vi "Enter.vi"(8 "error in (no error)":errorcluster, 10 "User Input":string, 11 "ATM Controller in":refnum<class "ATM Controller.lvclass">) -> (0 "error out":errorcluster, 3 "ATM Controller out":refnum<class "ATM Controller.lvclass">)   [LabVIEW 2020, in "ATM Controller.lvclass"]
uses:
  ATM Controller.lvclass
  ATM Controller.lvclass/ATM Controller.ctl
  Account Database/Account Database.lvclass
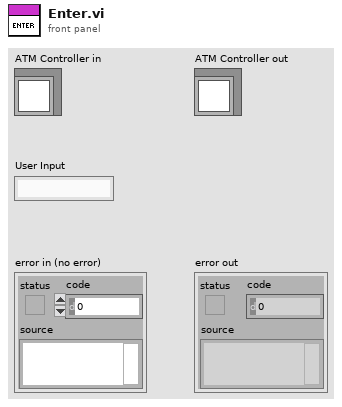
[diagram p1: front panel]
types:
  T1 = typedef "ATM Controller.lvclass/State.ctl" = enum16{"Start", "Card Inserted", "Verification Failed", "Verification Succeeded", "Terminate"}
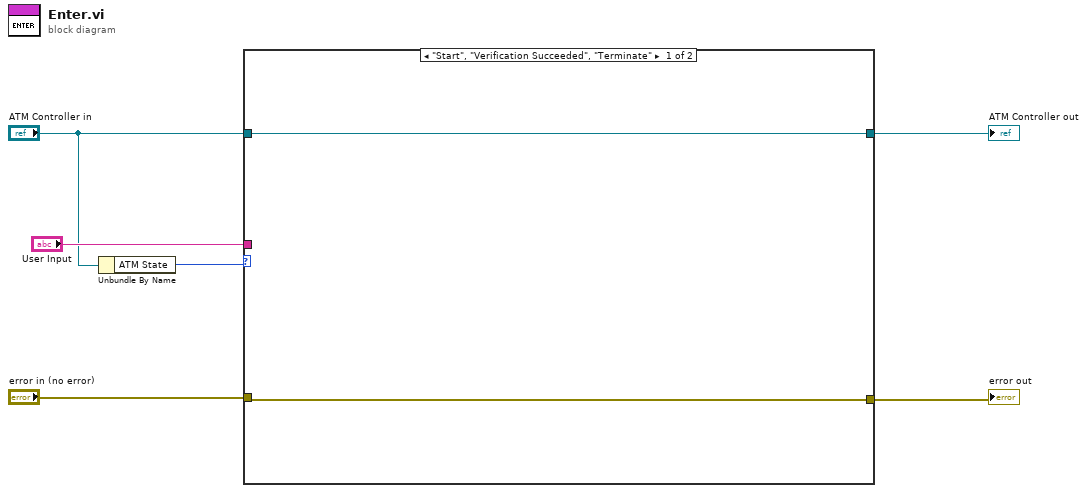
[diagram p0: block diagram]
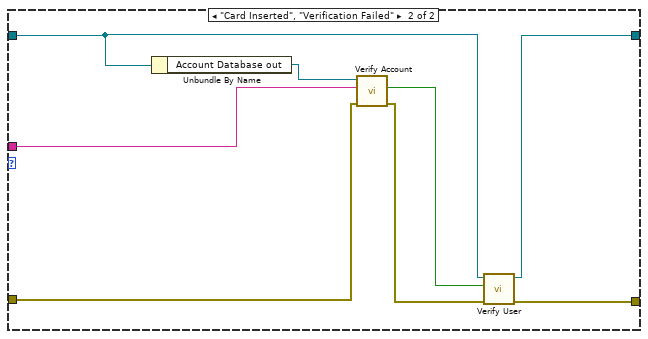
[diagram p2: hidden frame]
diagram:
  n1 = Unbundle By Name("ATM Controller in") -> ("ATM State"=w1:T1)
  n2 = case shown="\"Start\", \"Verification Succeeded\", \"Terminate\"" w1 {
    tunnel: "User Input" -> [_ w13]
    tunnel: [w7 w12] -> w5
    tunnel: "error in (no error)" -> [w7 w11]
    tunnel: "ATM Controller in" -> [w8 w10]
    tunnel: [w8 w9] -> w3
    frame "Start", "Verification Succeeded", "Terminate" {
    }
    frame "Card Inserted", "Verification Failed" {
      n3 = Unbundle By Name(w10) -> ("Account Database out"=w14:refnum<class "Account Database.lvclass">)
      n4 = call "Verify Account.vi"("error in (no error)"=w11, "Account Number"=w13, "Account Database in"=w14) -> ("error out"=w16:errorcluster, "Valid Account Number?"=w15:bool)  [unwired: 6 in, 1 out]
      n5 = call "Verify User.vi"("error in (no error)"=w16, "Verified?"=w15, "ATM Controller in"=w10) -> ("error out"=w12:errorcluster, "ATM Controller out"=w9:refnum<class "ATM Controller.lvclass">)  [unwired: 7 in]
    }
  }
  "error out" <- w5
  "ATM Controller out" <- w3
